vi "ResonanceAnalyzer.vi"() -> ()   [LabVIEW 2015]
uses:
  <vilib>/imath/engines/lvmath2/RunTimeEngine/Managers/WorkSpace/UID Generator.vi
  <vilib>/imath/engines/lvmath2/RunTimeEngine/RangeToken/NIMS_Range.vi
  <instcachedir>/0/NIMS_Range_D919CC09935940E88F755EC1C6F49AC1.lvgen/NIMS_Range_D919CC09935940E88F755EC1C6F49AC1_000.vi
  <vilib>/imath/engines/lvmath2/RunTimeEngine/RunTimeType/NIMS_RunTimeType_From StrictType (excl LVString).vi
  <instcachedir>/0/NIMS_RunTimeType_From StrictType (excl LVString)_EB1C38A9BC5048DA9ABDA8F781E54D21.lvgen/NIMS_RunTimeType_From StrictType (excl LVString)_EB1C38A9BC5048DA9ABDA8F781E54D21_000.vi
  <vilib>/imathl/engines/lvmath/Functions/Error Handling/Create Error.vi
  <vilib>/imath/engines/lvmath2/RunTimeEngine/LocalVariableDefStatement/MC_LocalVariableDefStatement_Display.vi
  <vilib>/imath/engines/lvmath2/RunTimeEngine/BuiltInFunctions/size/NIMS_I32Row=size(GRow).vi
  <instcachedir>/0/NIMS_I32Row=size(GRow)_E5C05C6B13124B29B774CC4F993D3C59.lvgen/NIMS_I32Row=size(GRow)_E5C05C6B13124B29B774CC4F993D3C59_000.vi
  <vilib>/imath/engines/lvmath2/RunTimeEngine/ArithmeticOperatorToken/NIMS_ArithmeticOperator_minus.vi
  <instcachedir>/0/NIMS_ArithmeticOperator_minus_8228ED1EA52B4CB8A68367813E4B0C9D.lvgen/NIMS_ArithmeticOperator_minus_8228ED1EA52B4CB8A68367813E4B0C9D_003.vi
  <vilib>/imath/engines/lvmath2/RunTimeEngine/IndexRead/NIMS M(S,S).vi
  <instcachedir>/0/NIMS M(S,S)_AC51E74150A542F7991B9634C66F3096.lvgen/NIMS M(S,S)_AC51E74150A542F7991B9634C66F3096_002.vi
  <vilib>/imath/engines/lvmath2/RunTimeEngine/BuiltInFunctions/randnormal/NIMS_randnormal(1,I32).vi
  <vilib>/imath/engines/lvmath2/RunTimeEngine/ErrorHandling/NIMS_Error From Error Code.vi
  <vilib>/imath/engines/lvmath2/RunTimeEngine/ArithmeticOperatorToken/NIMS_ArithmeticOperator_plus.vi
  <instcachedir>/0/NIMS_ArithmeticOperator_plus_A4F2756F5ADB4A0090E0DBD7C10701C8.lvgen/NIMS_ArithmeticOperator_plus_A4F2756F5ADB4A0090E0DBD7C10701C8_000.vi
  <vilib>/imath/engines/lvmath2/RunTimeEngine/Managers/SymbolTable/Clear UID.vi
  <vilib>/imath/engines/lvmath2/RunTimeEngine/NodeEndStatement/NIMS_NodeEndStatement_Output.vi
  <instcachedir>/0/NIMS_NodeEndStatement_Output_53EC0D466D134D7ABD903AC30B43404B.lvgen/NIMS_NodeEndStatement_Output_53EC0D466D134D7ABD903AC30B43404B_000.vi
  <instcachedir>/0/NIMS_NodeEndStatement_Output_53EC0D466D134D7ABD903AC30B43404B.lvgen/NIMS_NodeEndStatement_Output_53EC0D466D134D7ABD903AC30B43404B_005.vi
  <vilib>/imath/engines/lvmath2/RunTimeEngine/ErrorHandling/NIMS_Finalize Error.vi
  <vilib>/Utility/file.llb/Read Delimited Spreadsheet (DBL).vi
  <vilib>/imath/engines/lvmath2/RunTimeEngine/Managers/SymbolTable/NIMS_WorkSpace.lvlib
panel:
  out "Results":T1={"Amplitude"=0.4981819244631171, "Q"=-4.9403933423377895, "Center Frequency"=522.4440626994992}
  out "Resonance Curve":T2(graph)=[{"Best Gaussian Fit"=[10.0, 111.0, 212.0, 313.0, 414.0, 515.0, 615.0, 716.0, 817.0, 918.0, 1019.0, 1120.0, 1221.0, 1322.0, 1423.0, 1524.0, 1625.0, 1725.0, 1826.0, 1927.0, 2028.0, 2129.0, 2230.0, 2331.0, 2432.0, 2533.0, 2634.0, 2735.0, 2835.0, 2936.0, 3037.0, 3138.0, 3239.0, 3340.0, 3441.0, 3542.0, 3643.0, 3744.0, 3845.0, 3945.0, 4046.0, 4147.0, 4248.0, 4349.0, 4450.0, 4551.0, 4652.0, 4753.0, 4854.0, 4955.0, 5055.0, 5156.0, 5257.0, 5358.0, 5459.0, 5560.0, 5661.0, 5762.0, 5863.0, 5964.0, 6065.0, 6165.0, 6266.0, 6367.0, 6468.0, 6569.0, 6670.0, 6771.0, 6872.0, 6973.0, 7074.0, 7175.0, 7275.0, 7376.0, 7477.0, 7578.0, 7679.0, 7780.0, 7881.0, 7982.0, 8083.0, 8184.0, 8285.0, 8385.0, 8486.0, 8587.0, 8688.0, 8789.0, 8890.0, 8991.0, 9092.0, 9193.0, 9294.0, 9395.0, 9495.0, 9596.0, 9697.0, 9798.0, 9899.0, 10000.0], "all rows"=[0.0022156440963128597, 0.002289549302828971, 0.0019835812754562887, 0.030842530295634187, 0.06230888790580067, 0.5240225787620905, 0.10187086644722602, 0.1699417162886751, 0.16668633588877493, 0.08681604556119941, 0.3428467208333133, 0.07331620890272113, 0.0640324324468947, 0.20672833175376096, 0.042300938221809026, 0.0725103497617198, 0.05391380704697852, 0.032583670100200884, 0.25977658302294243, 0.02860882360627206, 0.03417432930562995, 0.059614238398731194, 0.02252163936956303, 0.05667610549418499, 0.02608254708161878, 0.020611044454724888, 0.17052968899095883, 0.018531048811186716, 0.024598011487888528, 0.03635381560138095, 0.015527445014329986, 0.04281539943374177, 0.019455840623720064, 0.015615288052686792, 0.1261101377297823, 0.014290584754776955, 0.019122734705510215, 0.030008894727241272, 0.012762918618217904, 0.036601594055804924, 0.016666714651981378, 0.014682499678319857, 0.08772027812959948, 0.0139331720528296, 0.02162718523727021, 0.02496605943079415, 0.014205286590397243, 0.05674792681823314, 0.018011504876186354, 0.01732207840428825, 0.07509309424540643, 0.01776028783647484, 0.026736219619997954, 0.03493815763832921, 0.017274281796735333, 0.04113391061524547, 0.024785632153941955, 0.017370007261373763, 0.0740542520651676, 0.019015160697745823, 0.017526693824662033, 0.07213565838990856, 0.013946010890131866, 0.01985409062924557, 0.026037542989387357, 0.011309671744302523, 0.029376496519615308, 0.013778438433514532, 0.010778293362395405, 0.0510093747291922, 0.009415643355550233, 0.012375136557590092, 0.01774393753761374, 0.008267039258319881, 0.02089055605593764, 0.01006352199189991, 0.008603992041441789, 0.03887764949279994, 0.00791589454624261, 0.01070286382911385, 0.020977319843964438, 0.007349368100487516, 0.012521316693126687, 0.01140512370007243, 0.006508036799845255, 0.019166817161706935, 0.007645396264150442, 0.0063694216537770925, 0.0241018289527433, 0.005795621301763043, 0.007144140713810944, 0.011213727544254225, 0.005201756278074573, 0.010209394837076797, 0.006692679069358428, 0.011946756171299781, 0.01768682993715307, 0.005365373995198518, 0.005717418729175535, 0.013989429371781666]}, {"Best Gaussian Fit"=[10.0, 111.0, 212.0, 313.0, 414.0, 515.0, 615.0, 716.0, 817.0, 918.0, 1019.0, 1120.0, 1221.0, 1322.0, 1423.0, 1524.0, 1625.0, 1725.0, 1826.0, 1927.0, 2028.0, 2129.0, 2230.0, 2331.0, 2432.0, 2533.0, 2634.0, 2735.0, 2835.0, 2936.0, 3037.0, 3138.0, 3239.0, 3340.0, 3441.0, 3542.0, 3643.0, 3744.0, 3845.0, 3945.0, 4046.0, 4147.0, 4248.0, 4349.0, 4450.0, 4551.0, 4652.0, 4753.0, 4854.0, 4955.0, 5055.0, 5156.0, 5257.0, 5358.0, 5459.0, 5560.0, 5661.0, 5762.0, 5863.0, 5964.0, 6065.0, 6165.0, 6266.0, 6367.0, 6468.0, 6569.0, 6670.0, 6771.0, 6872.0, 6973.0, 7074.0, 7175.0, 7275.0, 7376.0, 7477.0, 7578.0, 7679.0, 7780.0, 7881.0, 7982.0, 8083.0, 8184.0, 8285.0, 8385.0, 8486.0, 8587.0, 8688.0, 8789.0, 8890.0, 8991.0, 9092.0, 9193.0, 9294.0, 9395.0, 9495.0, 9596.0, 9697.0, 9798.0, 9899.0, 10000.0], "all rows"=[0.0019308232516655267, 0.022414554901059317, 0.048749558039092845, 0.09259569489052684, 0.19722526890485728, 0.4932473891624769, 0.26182538494030305, 0.15005299484415155, 0.1065675604806524, 0.08367404949963435, 0.06945165807491317, 0.059686425519461905, 0.052522520175969714, 0.04701545803374497, 0.04263296891872235, 0.03905149800881457, 0.03606253501100204, 0.03354858181625062, 0.031361358952326474, 0.029456482348658896, 0.027780827612462786, 0.026294070208201542, 0.024965005405666568, 0.02376907730303989, 0.022686675742062866, 0.02170193521251779, 0.020801870386362116, 0.019975742559325643, 0.01922183099523874, 0.018517567583673816, 0.017864388291023398, 0.017256816331076452, 0.01669014321794082, 0.016160296985314494, 0.015663736873406407, 0.01519736844149619, 0.014758474598264805, 0.014344659149875871, 0.01395380027535434, 0.013587575554403515, 0.01323699098860346, 0.01290430273354469, 0.012588157243811017, 0.012287335596442604, 0.012000737006930105, 0.011727364727809594, 0.01146631393502571, 0.011216761280656946, 0.010977955848947642, 0.01074921129923998, 0.010532026109056953, 0.010321484211159587, 0.010119272345451766, 0.009924901581908924, 0.009737920809887082, 0.00955791312612189, 0.009384492631384345, 0.009217301582573006, 0.00905600785483408, 0.00890030267484088, 0.008749898591859226, 0.008605943131208318, 0.008465309079414368, 0.008329226646528364, 0.00819747706781959, 0.008069855454048877, 0.007946169702991715, 0.00782623951231264, 0.007709895482903735, 0.007596978303121277, 0.007487338005497684, 0.007380833288497005, 0.007278341371897757, 0.0071776876418329656, 0.007079792787637982, 0.006984544413092886, 0.006891836170886983, 0.006801567359517585, 0.00671364255211632, 0.0066279712542813545, 0.006544467588296377, 0.006463050001384937, 0.00638364099588579, 0.006306924696899459, 0.006231297220485914, 0.006157468400253494, 0.006085374605981441, 0.006014955183532346, 0.005946152282335258, 0.005878910694766322, 0.00581317770647805, 0.005748902956813964, 0.005686038308522512, 0.005624537726053543, 0.005564946677507926, 0.005506031514098513, 0.005448354209846687, 0.005391876052600728, 0.005336559931944506, 0.005282370257000198]}]
  in  "?":enum32{"Simulation", "Experiment"}(tab)=enum."Experiment"
  in  "Input Parameters":T3={"Q"=10.0, " Center Frequency"=600.0, " Start Frequency"=400.0, "End Frequency"=800.0, " dF"=5.0, " Noise Level"=0.01}
  in  "Path":path=path "C:/Users/Brian/Desktop/New folder/week6/Spreadsheet"
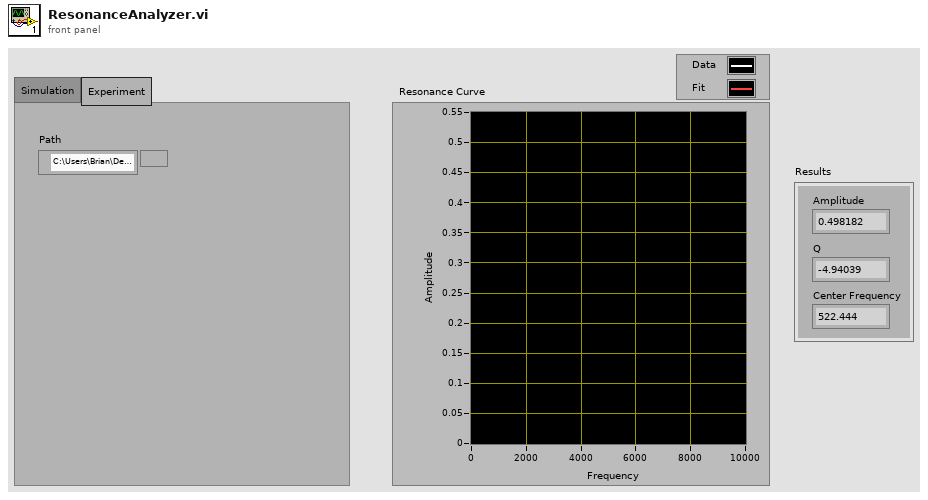
[diagram p1: front panel]
types:
  T1 = cluster{"Amplitude":dbl, "Q":dbl, "Center Frequency":dbl}
  T2 = cluster{"Best Gaussian Fit":dbl[], "all rows":dbl[]}[]
  T3 = cluster{"Q":dbl, " Center Frequency":dbl, " Start Frequency":dbl, "End Frequency":dbl, " dF":dbl, " Noise Level":dbl}
  T4 = cluster{"Array[0]":dbl, "Array[1]":dbl, "Array[2]":dbl, "Array[3]":dbl, "Array[4]":dbl, "Array[5]":dbl, "Array[6]":dbl, "Array[7]":dbl, "Array[8]":dbl}
  T5 = cluster{"Array[2]":dbl, "Array[0]":dbl, "Array[1]":dbl}
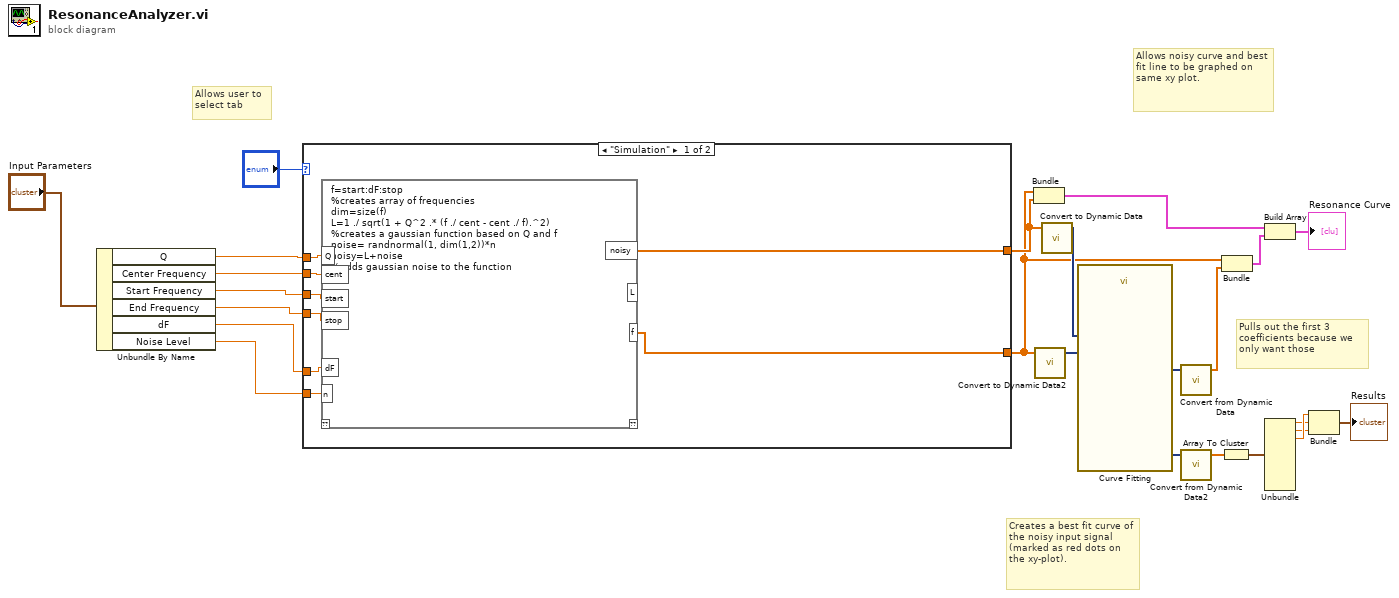
[diagram p0: block diagram]
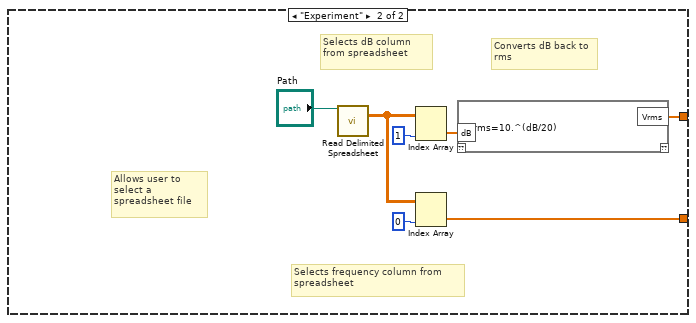
[diagram p2: hidden frame]
diagram:
  # "Allows noisy curve and best fit line to be graphed on same xy plot."
  # "Pulls out the first 3 coefficients because we only want those"
  # "Creates a best fit curve of the noisy input signal (marked as red dots on the xy-plot)."
  # "Allows user to select tab"
  n1 = Unbundle By Name("Input Parameters") -> ("Q"=w22:dbl, "Center Frequency"=w21:dbl, "Start Frequency"=w20:dbl, "End Frequency"=w19:dbl, "dF"=w18:dbl, "Noise Level"=w15:dbl)
  n2 = case shown="\"Simulation\"" "?" {
    tunnel: w22 -> [w28 _]
    tunnel: w21 -> [w29 _]
    tunnel: w20 -> [w32 _]
    tunnel: w19 -> [w31 _]
    tunnel: w18 -> [w30 _]
    tunnel: [w27 w215] -> w8
    tunnel: [w25 w214] -> w10
    tunnel: w15 -> [w26 _]
    frame "Simulation" {
      n3 = mathscript code="f=start:dF:stop\n%creates array of frequencies\ndim=size(f)\nL=1 ./ sqrt(1 + Q^2 .* (f ./ cent - cent ./ f).^2)\n%creates a gaussian function based on Q and f\nnoise= randnormal(1, dim(1,2))*n\nnoisy=L+noise\n%adds gaussian noise to the function"("start"=w32, "stop"=w31, "dF"=w30, "cent"=w29, "Q"=w28, "n"=w26) -> ("f"=w27:dbl[], "noisy"=w25:cdb[])  [unwired: 1 in, 2 out]
    }
    frame "Experiment" {
      # "Selects frequency column from spreadsheet"
      # "Selects dB column from spreadsheet"
      # "Converts dB back to rms"
      # "Allows user to select a spreadsheet file"
      n4 = call-poly <vilib>:"Read Delimited Spreadsheet.vi"("file path (dialog if empty)"="Path") -> ("all rows"=w220:dbl[][])  [unwired: 9 in, 5 out]
      n5 = Index Array(array=w220, index (col)=1) -> (element=w217:dbl[])  [unwired: 1 in]
      n6 = Index Array(array=w220, index (col)=0) -> (element=w215:dbl[])  [unwired: 1 in]
      n7 = mathscript code="Vrms=10.^(dB/20)"("dB"=w217) -> ("Vrms"=w214:dbl[])  [unwired: 1 in, 1 out]
    }
  }
  n8 = Bundle("all rows"=w8, "noisy"=w10) -> (w17:cluster{"all rows":dbl[], "noisy":cdb[]})  [unwired: 1 in]
  n9 = call "Convert to Dynamic Data2"("Array"=w8) -> ("Dynamic Data Type"=w12:dynamicdata)  [unwired: 3 in]
  n10 = call "Convert to Dynamic Data"("Array"=w10) -> ("Dynamic Data Type"=w14:dynamicdata)  [unwired: 3 in]
  n11 = call "Curve Fitting"("Locations"=w12, "Signals"=w14) -> ("best fit"=w13:dynamicdata, "non-linear coefficients"=w11:dynamicdata)  [unwired: 5 in, 3 out]
  n12 = call "Convert from Dynamic Data"("Dynamic Data Type"=w13) -> ("Array"=w9:dbl[])  [unwired: 3 in]
  n13 = call "Convert from Dynamic Data2"("Dynamic Data Type"=w11) -> ("Array"=w6:dbl[])  [unwired: 3 in]
  n14 = Array To Cluster(array=w6) -> (cluster=w5:T4)
  n15 = Bundle("all rows"=w8, "Array"=w9) -> (w7:cluster{"all rows":dbl[], "Array":dbl[]})  [unwired: 1 in]
  n16 = Build Array(w17, w7) -> (→"Resonance Curve":cluster{"all rows":dbl[], "noisy":cdb[]}[])
  n17 = Unbundle(w5) -> ("Array[0]"=w2:dbl, "Array[1]"=w1:dbl, "Array[2]"=w3:dbl)  [unwired: 6 out]
  n18 = Bundle("Array[2]"=w3, "Array[0]"=w2, "Array[1]"=w1) -> (→"Results":T5)  [unwired: 1 in]
